vi "updateB.vi"(6 "B [T] new":dbl, 11 "MagAnalysis_Online in":refnum<class "MagAnalysis_Online.lvclass">) -> (3 "MagAnalysis_Online out":refnum<class "MagAnalysis_Online.lvclass">)   [LabVIEW 2013, in "MagAnalysis_Online.lvclass"]
uses:
  MagAnalysis_Online.lvclass
  MagAnalysis_Online.lvclass/MagAnalysis_Online.ctl
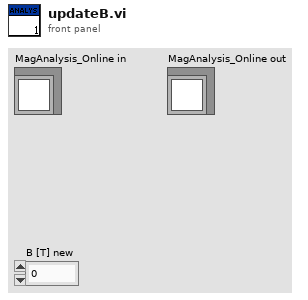
[diagram p1: front panel]
types:
  T1 = typedef "Calib_Typdef.ctl" = cluster{"cam 0":T2, "cam 1":T2, "cam 2":T2, "cam 3":T2}
  T2 = typedef "calib_Sub_Typdef.ctl" = cluster{"incident ANGLE COMPENSATION":dbl[], "dp/B [MeV/C/B]":dbl[], "charge compensation":dbl[], "Momentum [MeV/C]":dbl[], "energyDependence Input":dbl[], "pixel angle (y)":dbl[], "dp [MeV/C/] ":dbl[], "angle 2Dfor spectrumj":dbl[][], "dp [MeV/C] 2D":dbl[][], "charge compensation 2D":dbl[][], "Screen&Camera 2":T3, "ROI info":T5, "Y 2D full angle":dbl[][], "calib pixel":T6, "2D":T7, "UserROI":T8, "final":T9, "B[T]":dbl, "index":dbl}
  T3 = typedef "ScreenCam2_TypDEf.ctl" = cluster{"Screen Orientation":string, "Screen angle":string, "Lens":T4, "Calibration (mm/pix)":dbl}
  T4 = typedef "CamAndObj_TypDEf.ctl" = enum16{"FL1-f8x08", "FL1-f8x06", "FL1-f8", "ch300-f50", "FL2G-f8", "FL3M14-f8", "FL3M14-f8x08", "FL3M14-f8x08(2x2)"}
  T5 = typedef "ROIInfo_TypDef.ctl" = cluster{"npix-X":i32, "npix-Y":i32, "Left [pix]":dbl, "Top [pix]":dbl}
  T6 = typedef "calibPixel.ctl" = cluster{"y1(pixel)":dbl[], "y2(pixel)":dbl[], "dp/B [MeV/C/B] (pixel)":dbl[], "energyDependence Input(pixel)":dbl[], "bending angle [deg](pixel)":dbl[], "total path(pixel)":dbl[], "pixel angle (y)(pixel)":dbl[], "energy dependence (pixel)":dbl[], "charge compensation (pixel)":dbl[], "Momentum [MeV/C](pixel)":dbl[], "angular compensation(pixel)":dbl[]}
  T7 = typedef "2DTypDef.ctl" = cluster{"dp":dbl[][], "chargeCompensation":dbl[][], "angle":dbl[][], "Momentum":dbl[][]}
  T8 = typedef "CamRoiTypDef.ctl" = cluster{"Width":dbl, "Hight":dbl, "OffsetX":dbl, "OffsetY":dbl}
  T9 = typedef "finalCalibTypdef.ctl" = cluster{"X":dbl[][], "xi":dbl[][], "delta momentum":dbl, "Y":dbl[][], "yi":dbl[][], "angle (Y)":dbl[], "delta angle":dbl, "scale delta angle":dbl, "intraX":dbl, "intraY":dbl, "mask":dbl[][]}
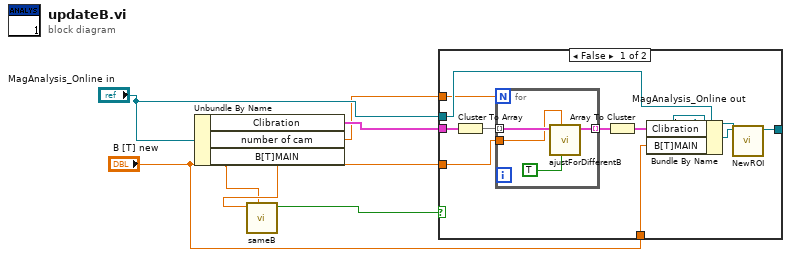
[diagram p0: block diagram]
diagram:
  n1 = Unbundle By Name("MagAnalysis_Online in") -> ("Clibration"=w5:T1, "number of cam"=w3:dbl, "B[T]MAIN"=w2:dbl)
  n2 = call "sameB.vi"("B [T] new"="B [T] new", "B [T] old"=w2) -> ("Boolean"=w4:bool)  [unwired: 9 in]
  n3 = case shown="False" w4 {
    tunnel: w5 -> [w17 _]
    tunnel: "B [T] new" -> [w15 _]
    tunnel: "MagAnalysis_Online in" -> [w12 w22]
    tunnel: [w14 w22] -> w7
    tunnel: w3 -> [w9 _]
    tunnel: "B [T] new" -> [w8 _]
    frame False {
      n4 = Cluster To Array(cluster=w17) -> (array=w16:T2[])
      n5 = for {
        N: w9 -> [_]
        tunnel: w16 -> [w21] mode=indexing
        tunnel: w15 -> [w20]
        tunnel: [w19] -> w13 mode=indexing
        n6 = call "ajustForDifferentB.vi"("force (FALSE)"=TRUE, "B [T]"=w20, "Cam Cluster out in"=w21) -> ("Cam Cluster out out"=w19:T2)  [unwired: 7 in, 1 out]
      }
      n7 = Array To Cluster(array=w13) -> (cluster=w11:cluster{"[0]":T2, "[1]":T2, "[2]":T2, "[3]":T2})
      n8 = Bundle By Name(cluster=w12, "Clibration"=w11, "B[T]MAIN"=w8) -> (w10:refnum<class "MagAnalysis_Online.lvclass">)
      n9 = call "NewROI.vi"("MagAnalysis_Online in"=w10) -> ("MagAnalysis_Online out"=w14:refnum<class "MagAnalysis_Online.lvclass">)  [unwired: 10 in]
    }
    frame True {
    }
  }
  "MagAnalysis_Online out" <- w7
